vi "King Swap.vi"(0 "1D Board":T1[](array[typedef]), 5 "DT Team #":i32, 11 "error in (no error)":errorcluster) -> (4 "1D Board Out":T1[](array[typedef]), 6 "Cell to move to":i32, 8 "Output Text":string, 15 "error out":errorcluster)   [LabVIEW 2014, in "Dragon Tamers.lvlib"]
uses:
  Dragon Tamers.lvlib
  Typedefs/Board Cell.ctl
  Typedefs/Cell Occupancy.ctl
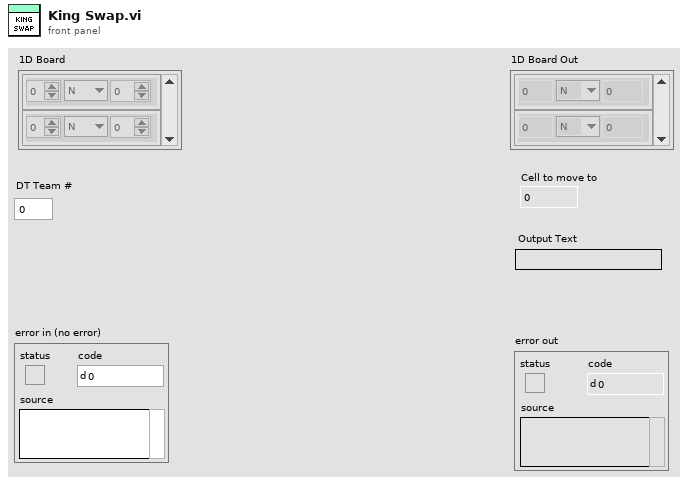
[diagram p1: front panel]
types:
  T1 = typedef "Dragon Tamers.lvlib/Board Cell.ctl" = cluster{"Team":i32, "Occu.":T2, "Count":i32}
  T2 = typedef "Dragon Tamers.lvlib/Cell Occupancy.ctl" = enum16{"N", "C", "K"}
  T3 = typedef "Dragon Tamers.lvlib/Parsed Board.ctl" = cluster{"DT King":i32, "Opp King":i32, "Count":i32[], "Empty Cells":i32[], "DT Cells":i32[], "Opp Cells":i32[], "DT Team":i32, "Opp. Team":i32}
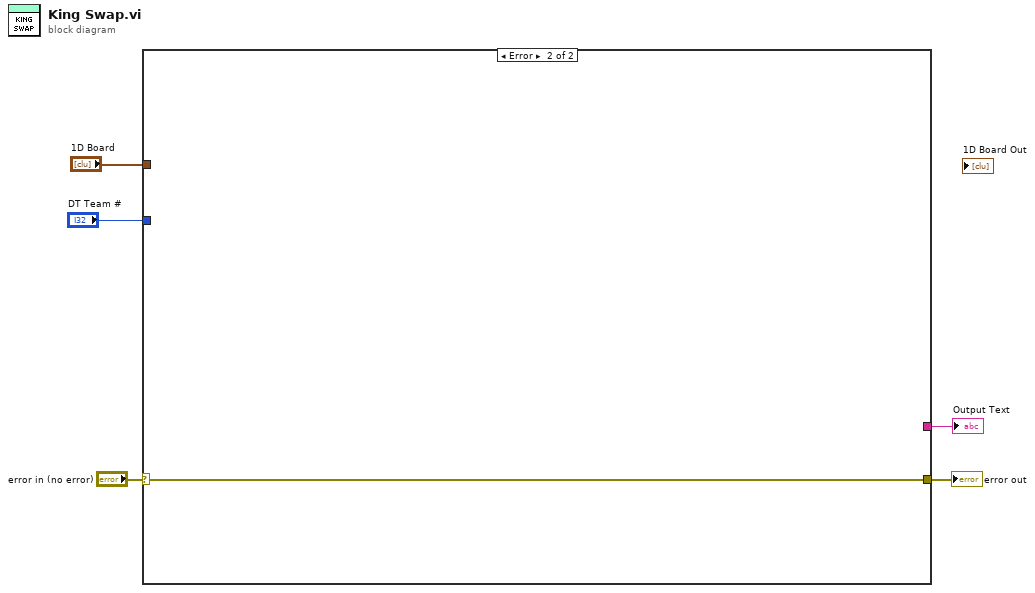
[diagram p0: block diagram]
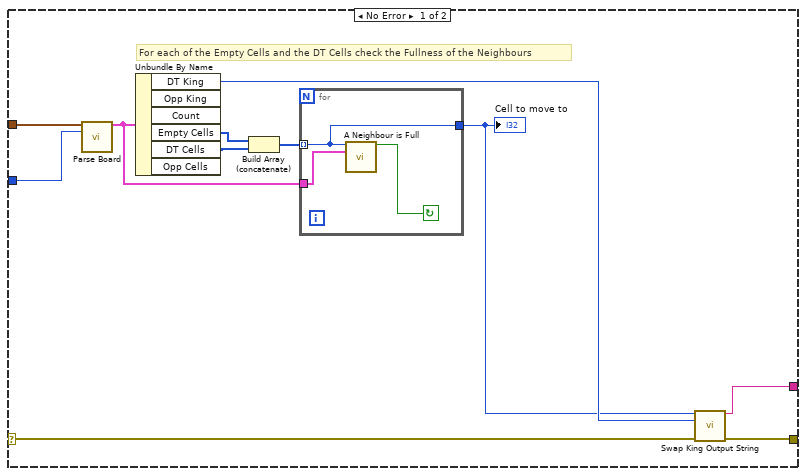
[diagram p2: hidden frame]
diagram:
  n1 = case shown="Error" "error in (no error)" {
    selector: "error in (no error)" -> [w7 w20]
    tunnel: [w14 w20] -> w4
    tunnel: "1D Board" -> [w16 _]
    tunnel: "DT Team #" -> [w15 _]
    tunnel: [w6 _] -> w1
    frame No Error {
      # "For each of the Empty Cells and the DT Cells check the Fullness of the Neighbours"
      n2 = call "Parse Board.vi"("Board Array"=w16, "DT Team #"=w15) -> ("Parsed Board Info"=w10:T3)  [unwired: 12 in, 1 out]
      n3 = Unbundle By Name(w10) -> ("DT King"=w9:i32, "Empty Cells"=w13:i32[], "DT Cells"=w12:i32[])  [unwired: 3 out]
      n4 = Build Array (concatenate)(w13, w12) -> (w11:i32[])
      n5 = for {
        tunnel: w11 -> [w17] mode=indexing
        tunnel: w10 -> [w19]
        tunnel: [w17] -> w8
        stop <- w18 continue-if-true
        n6 = call "A Neighbour is Full.vi"("Cell"=w17, "Parsed Board"=w19) -> ("Full?"=w18:bool)  [unwired: 12 in, 1 out]
      }
      "Cell to move to" <- w8
      n7 = call "Swap King Output String.vi"("New Cell Index"=w8, "Old Cell Index"=w9, "error in (no error)"=w7) -> ("Output Text"=w6:string, "error out"=w14:errorcluster)  [unwired: 11 in]
    }
    frame Error {
    }
  }
  "error out" <- w4
  "Output Text" <- w1
